vi "Labview_FLIR_A65_TCP.vi"() -> ()   [LabVIEW 2017]
uses:
  <vilib>/userdefined/High Color/IMAQdx.ctl
  <vilib>/vision/driver/NI_Vision_Acquisition_Software.lvlib
  <resource>/objmgr/imaqdx.rc
panel:
  in  "port":u16=3500
  in  "Ring":i64(ring)=17301505 items=["Mono 8"=17301505, "Mono14"=17825829, "Mono16"=17825799]
  in  "IRFormat":i64(ring)=2 items=["LowGainMode"=1, "HighGainMode"=2]
  in  "IRFrameRate":i64(ring) items=["NTSC30HZ"=0, "PAL25Hz"=1, "NTSC60HZ"=4, "PAL50HZ"=5]
  out "Image":T1(plugin-control)
  in  "Session In":T2="FLIR AX5"
  # "Please select the camera you want to access the thermal image and the parameters"
  # "Please select the port for TCP Connection"
  # "Note: The Image control needs to be set to 8-bit display. This is done by with the following steps\n            1) Right click on the Image display and select 8-Bit Display Mapping to bring up Set 8 Bit Display Mapping window\n            2) Un-tick \"Apply mapping only when Configured bit depth is 0\" in the Set 8 Bit Display Mapping window\n            3) Set the Conversion Method to Full Dynamic if not already selected"
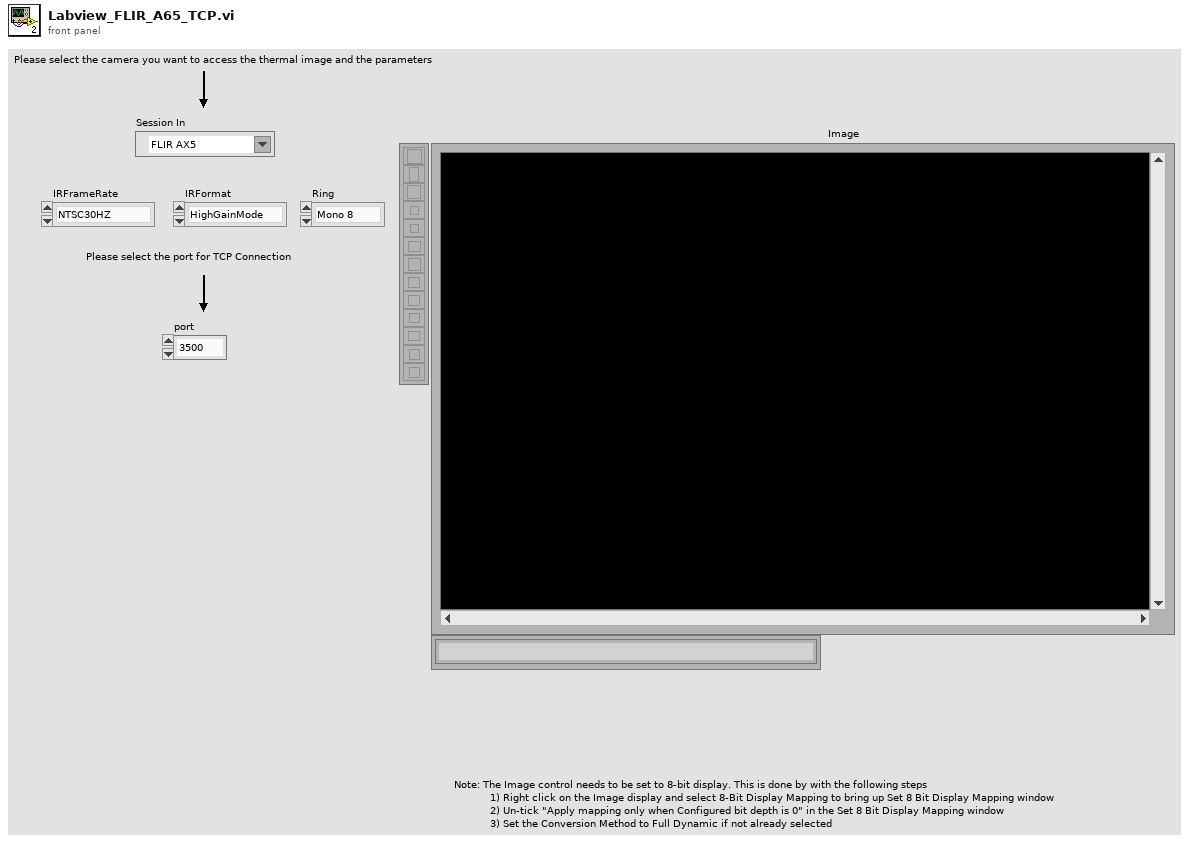
[diagram p1: front panel]
types:
  T1 = typedef "IMAQ Image.ctl" = refnum<image>
  T2 = typedef "IMAQdx.ctl" = refnum<k21>
  T3 = typedef "Image Type" = u32
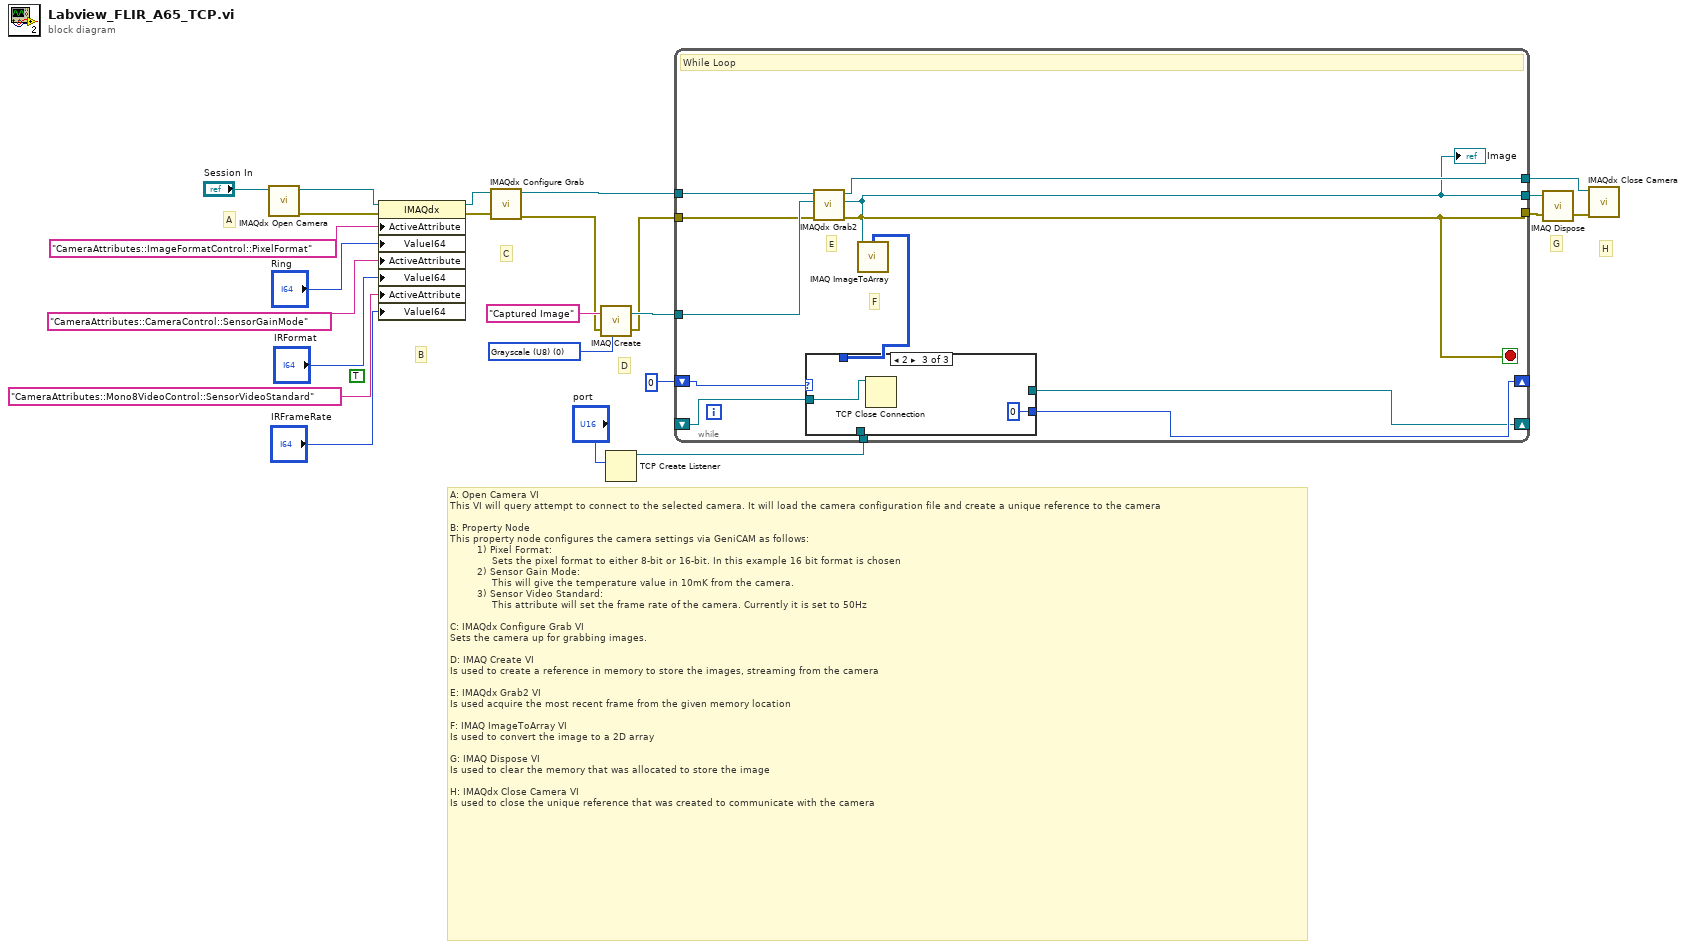
[diagram p0: block diagram]
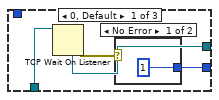
[diagram p2: hidden frame]
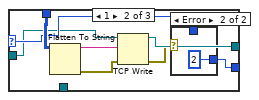
[diagram p4: hidden frame]
diagram:
  (unwired) TRUE ("ValueBool")
  w19 = T3 0 items=["Grayscale (U8)", "Grayscale (I16)", "Grayscale (SGL)", "Complex (CSG)", "RGB (U32)", "HSL (U32)", "RGB (U64)", "Grayscale (U16)"] ("Image Type")
  # "A: Open Camera VI\nThis VI will query attempt to connect to the selected camera. It will load the camera configuration file and create a unique reference to the camera\n\nB: Property Node\nThis property node configures the camera settings via GeniCAM as follows:\n         1) Pixel Format:\n              Sets the pixel format to either 8-bit or 16-bit. In this example 16 bit format is chosen\n         2) Sensor Gain Mode:\n              This will give the temperature value in 10mK from the camera.\n         3) Sensor Video Standard:\n              This attribute will set the frame rate of the camera. Currently it is set to 50Hz\n\nC: IMAQdx Configure Grab VI\nSets the camera up for grabbing images.\n\nD: IMAQ Create VI\nIs used to create a reference in memory to store the images, streaming from the camera\n\nE: IMAQdx Grab2 VI\nIs used acquire the most recent frame from the given memory location\n\nF: IMAQ ImageToArray VI\nIs used to convert the image to a 2D array\n\nG: IMAQ Dispose VI\nIs used to clear the memory that was allocated to store the image\n\nH: IMAQdx Close Camera VI\nIs used to close the unique reference that was created to communicate with the camera"
  # "H"
  # "G"
  # "D"
  # "C"
  # "B"
  # "A"
  n1 = call <vilib>:"IMAQdx Open Camera.vi"("Session In"="Session In") -> ("error out"=w23:errorcluster, "Session Out"=w16:T2)  [unwired: 9 in]
  n2 = property class="IMAQdx"(reference=w16, error in=w23, "ActiveAttribute"="CameraAttributes::ImageFormatControl::PixelFormat", "ValueI64"="Ring", "ActiveAttribute"="CameraAttributes::CameraControl::SensorGainMode", "ValueI64"="IRFormat", "ActiveAttribute"="CameraAttributes::Mono8VideoControl::SensorVideoStandard", "ValueI64"="IRFrameRate") -> (reference out=w22:T2, error out=w12:errorcluster)
  n3 = call <vilib>:"IMAQdx Configure Grab.vi"("error in"=w12, "Session In"=w22) -> ("error out"=w11:errorcluster, "Session Out"=w21:T2)  [unwired: 8 in]
  n4 = call "IMAQ Create"("Image Name"="Captured Image", "Image Type"=w19, "error in (no error)"=w11) -> ("New Image"=w18:T1, "error out"=w10:errorcluster)  [unwired: 2 in]
  n5 = TCP Create Listener(10:"port") -> (3:w5:refnum<k5>)  [unwired: 4 in, 2 out]
  n6 = while {
    tunnel: w10 -> [w33]
    tunnel: w21 -> [w36]
    tunnel: w18 -> [w34]
    tunnel: [w35] -> w17
    tunnel: w5 -> [w32]
    shift-right: [w30] -> _
    shift-left: 0 -> [w31]
    shift-right: [w28] -> _
    shift-left: _ -> [w29]
    tunnel: [w27] -> w2
    tunnel: [w25] -> w1
    stop <- w25 stop-if-true
    # "F"
    # "E"
    # "While Loop"
    n7 = call <vilib>:"IMAQdx Grab2.vi"("error in"=w33, "Image In"=w34, "Session In"=w36) -> ("error out"=w25:errorcluster, "Image Out"=w27:T1, "Session Out"=w35:T2)  [unwired: 5 in, 1 out]
    "Image" <- w27
    n8 = call "IMAQ ImageToArray"("error in (no error)"=w25, "Image"=w27) -> ("Image Pixels (U8)"=w26:u8[][])  [unwired: 2 in, 4 out]
    n9 = case shown="2" w31 {
      selector: w31 -> [_ w44 _]
      tunnel: w32 -> [w40 _ _]
      tunnel: [w39 w47 _] -> w28
      tunnel: [w37 w45 0] -> w30
      tunnel: w29 -> [_ w42 w53]
      tunnel: w26 -> [_ w49 _]
      frame 0, Default {
        n10 = TCP Wait On Listener(11:w40) -> (0:w38:errorcluster, 4:w39:refnum<k5>)  [unwired: 3 in, 3 out]
        n11 = case shown="No Error" w38 {
          tunnel: [1 _] -> w37
          frame No Error {
          }
          frame Error {
          }
        }
      }
      frame 1 {
        n12 = Flatten To String(anything=w49) -> (data string=w48:string, error out=w43:errorcluster)  [unwired: 3 in, 1 out]
        n13 = TCP Write(connection ID=w42, data in=w48, error in (no error)=w43) -> (connection ID out=w47:refnum<k5>, error out=w46:errorcluster)  [unwired: 1 in, 1 out]
        n14 = case shown="Error" w46 {
          tunnel: [w50 2] -> w45
          tunnel: w44 -> [w50 _]
          frame No Error {
          }
          frame Error {
          }
        }
      }
      frame 2 {
        n15 = TCP Close Connection(connection ID=w53) -> ()  [unwired: 2 in, 2 out]
      }
    }
  }
  n16 = call "IMAQ Dispose"("Image"=w2, "error in (no error)"=w1) -> ("error out"=w9:errorcluster)  [unwired: 4 in]
  n17 = call <vilib>:"IMAQdx Close Camera.vi"("error in"=w9, "Session In"=w17) -> ()  [unwired: 9 in, 1 out]
